vi "Subscribe to Results.vi"(8 "error in (no error)":errorcluster, 10 "Result Observer":refnum<class "Result Observer.lvclass">, 11 "Parallell Test Runner In":refnum<class "Parallell Test Runner.lvclass">) -> (0 "error out":errorcluster, 3 "Parallell Test Runner Out":refnum<class "Parallell Test Runner.lvclass">)   [LabVIEW 2020, in "Parallell Test Runner.lvclass"]
uses:
  Parallell Test Runner.lvclass
  Parallell Test Runner.lvclass/Parallell Test Runner.ctl
  Result Observer/Result Observer.lvclass
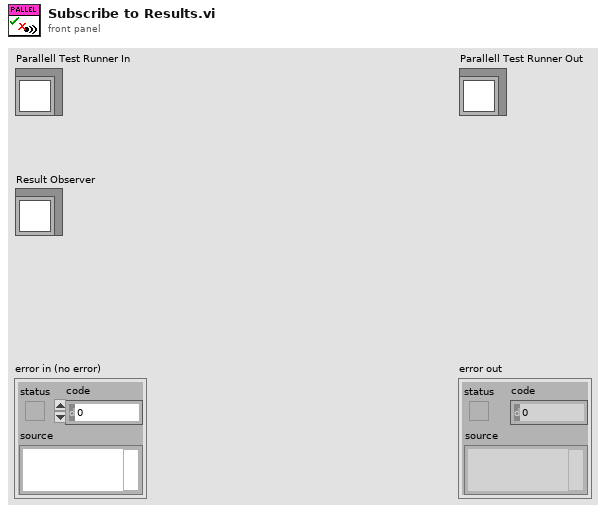
[diagram p1: front panel]
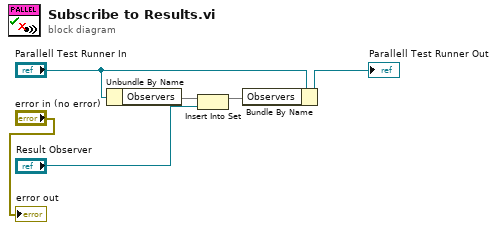
[diagram p0: block diagram]
diagram:
  n1 = Unbundle By Name("Parallell Test Runner In") -> ("Observers"=w3:set{refnum<class "Result Observer.lvclass">})
  n2 = Insert Into Set(10:"Result Observer", 11:w3) -> (3:w2:set{refnum<class "Result Observer.lvclass">})  [unwired: 1 out]
  n3 = Bundle By Name(cluster="Parallell Test Runner In", "Observers"=w2) -> (→"Parallell Test Runner Out":refnum<class "Parallell Test Runner.lvclass">)
  "error out" <- "error in (no error)"
